vi "Check Action.vi"(6 "HRS Time":dbl, 7 "Values In":dbl[](array[numeric]), 8 "error in (no error)":errorcluster, 11 "Valve in":refnum<class "TimedPWMControl.lvclass">) -> (0 "error out":errorcluster, 1 "Do Action":bool, 2 "Action":T1, 3 "Valve out":refnum<class "TimedPWMControl.lvclass">, 5 "Values":dbl[](array[numeric]))   [LabVIEW 2020, in "VolatusControl.lvlib" / "TimedPWMControl.lvclass"]
uses:
  TimedPWMControl.lvclass
  Valve Action.ctl
  Volatus/MessageQ/MessageQ.lvclass
  TimedPWMControl.lvclass/TimedPWMControl.ctl
  State.ctl
  lv-vecto/Vecto/Channel/Channel.lvclass/Channel.ctl
  lv-vecto/Vecto/Group/Value by Index.vi
  VolatusControl.lvlib
  lv-control/IG PID/PID/PID.lvclass
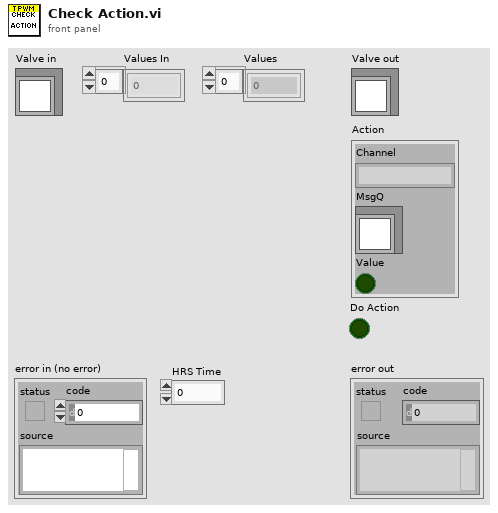
[diagram p1: front panel]
types:
  T1 = typedef "VolatusControl.lvlib/Valve Action.ctl" = cluster{"Channel":string, "MsgQ":refnum<class "MessageQ.lvclass">, "Value":bool}
  T2 = typedef "VolatusControl.lvlib/TimedPWMControl.lvclass/State.ctl" = enum16{"Idle", "Start", "Enabled", "Disable"}
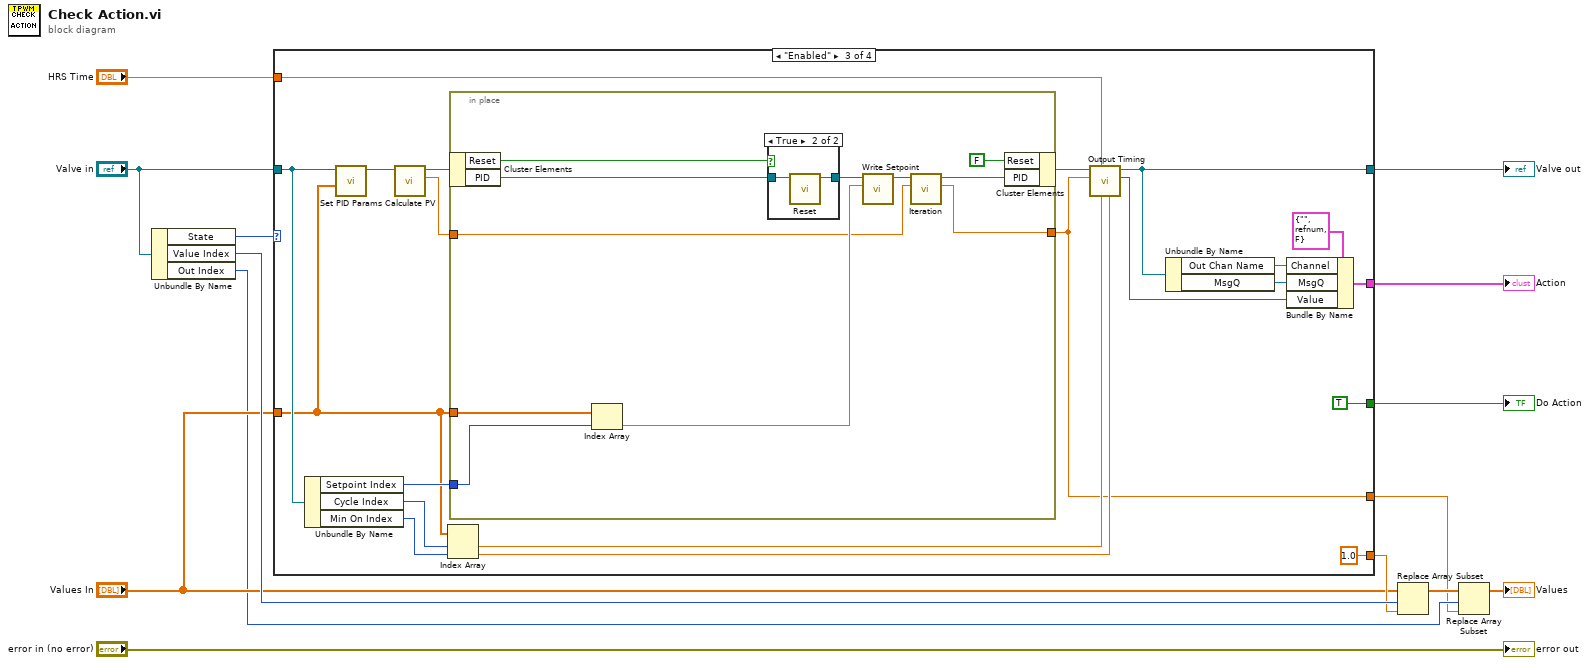
[diagram p0: block diagram]
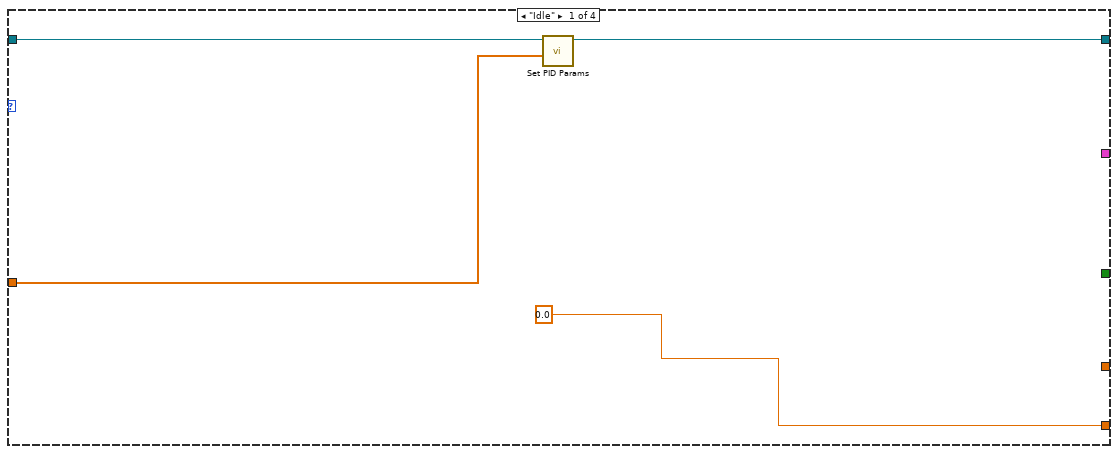
[diagram p2: hidden frame]
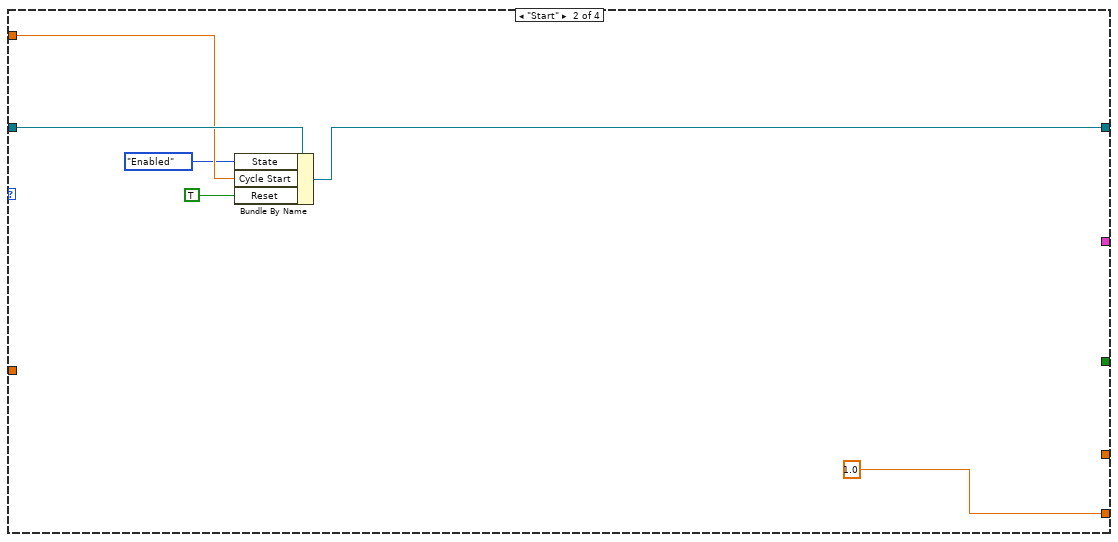
[diagram p3: hidden frame]
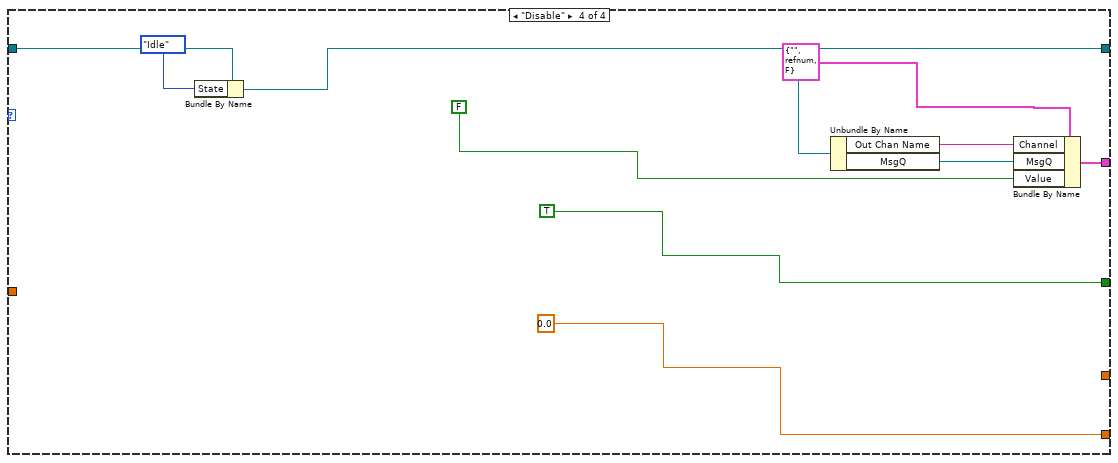
[diagram p5: hidden frame]
diagram:
  n1 = Unbundle By Name("Valve in") -> ("State"=w12:T2, "Value Index"=w13:i32, "Out Index"=w5:i32)
  n2 = case shown="\"Enabled\"" w12 {
    tunnel: [0.0 1.0 1.0 0.0] -> w11
    tunnel: [_ _ TRUE ("Do Action") TRUE ("Do Action")] -> w10
    tunnel: [_ _ w40 w67] -> w9
    tunnel: [w16 w21 w34 w61] -> w8
    tunnel: "Values In" -> [w15 _ w27 _]
    tunnel: [_ _ w31 _] -> w3
    tunnel: "HRS Time" -> [_ w23 w30 _]
    tunnel: "Valve in" -> [w17 w24 w29 w64]
    frame "Idle" {
      n3 = call "Set PID Params.vi"("Values"=w15, "TimedPWMControl in"=w17) -> ("TimedPWMControl out"=w16:refnum<class "TimedPWMControl.lvclass">)  [unwired: 8 in, 1 out]
    }
    frame "Start" {
      n4 = Bundle By Name(cluster=w24, "State"=State."Enabled", "Cycle Start"=w23, "Reset"=TRUE) -> (w21:refnum<class "TimedPWMControl.lvclass">)
    }
    frame "Enabled" {
      n5 = Unbundle By Name(w29) -> ("Setpoint Index"=w41:i32, "Cycle Index"=w39:i32, "Min On Index"=w38:i32)
      n6 = call "Set PID Params.vi"("Values"=w27, "TimedPWMControl in"=w29) -> ("TimedPWMControl out"=w28:refnum<class "TimedPWMControl.lvclass">)  [unwired: 8 in, 1 out]
      n7 = call "Calculate PV.vi"("TimedPWMControl in"=w28) -> ("PV"=w25:dbl, "TimedPWMControl out"=w26:refnum<class "TimedPWMControl.lvclass">)  [unwired: 8 in, 1 out]
      n8 = Index Array(array=w27, index #1=w39, index #2=w38) -> (element #1=w37:dbl, element #2=w36:dbl)
      n9 = in-place {
        in-place-border: w41 -> [w54]
        in-place-border: w27 -> [w55]
        in-place-border: [w51] -> w31
        in-place-border: w25 -> [w46]
        n10 = in-place-cluster #1(w26) -> ("Reset"=w48:bool, "PID"=w47:refnum<class "PID.lvclass">)
        n11 = Index Array(array=w55, index=w54) -> (element=w53:dbl)
        n12 = case shown="True" w48 {
          tunnel: w47 -> [w57 w59]
          tunnel: [w57 w58] -> w49
          frame False {
          }
          frame True {
            n13 = call "Reset.vi"("PID in"=w59) -> ("PID out"=w58:refnum<class "PID.lvclass">)  [unwired: 9 in, 1 out]
          }
        }
        n14 = call "Write Setpoint.vi"("Setpoint"=w53, "PID in"=w49) -> ("PID out"=w56:refnum<class "PID.lvclass">)  [unwired: 8 in, 1 out]
        n15 = call "Iteration.vi"("Process Value"=w46, "PID in"=w56) -> ("Output"=w51:dbl, "PID out"=w52:refnum<class "PID.lvclass">)  [unwired: 6 in, 2 out]
        n16 = in-place-cluster #1("Reset"=FALSE, "PID"=w52) -> (w42:refnum<class "TimedPWMControl.lvclass">)
      }
      n17 = call "Output Timing.vi"("Min On"=w36, "Cycle"=w37, "HRS Time"=w30, "Out 0-1"=w31, "TimedPWMControl in"=w42) -> ("Output"=w35:bool, "TimedPWMControl out"=w34:refnum<class "TimedPWMControl.lvclass">)  [unwired: 4 in, 1 out]
      n18 = Unbundle By Name(w34) -> ("Out Chan Name"=w33:string, "MsgQ"=w32:refnum<class "MessageQ.lvclass">)
      n19 = Bundle By Name(cluster=T1 {"Channel"="", "MsgQ"=refnum, "Value"=FALSE} ("Action"), "Channel"=w33, "MsgQ"=w32, "Value"=w35) -> (w40:T1)
    }
    frame "Disable" {
      n20 = Bundle By Name(cluster=w64, "State"=State."Idle") -> (w61:refnum<class "TimedPWMControl.lvclass">)
      n21 = Unbundle By Name(w61) -> ("Out Chan Name"=w62:string, "MsgQ"=w63:refnum<class "MessageQ.lvclass">)
      n22 = Bundle By Name(cluster=T1 {"Channel"="", "MsgQ"=refnum, "Value"=FALSE} ("Action"), "Channel"=w62, "MsgQ"=w63, "Value"=FALSE) -> (w67:T1)
    }
  }
  "Valve out" <- w8
  "Action" <- w9
  "Do Action" <- w10
  n23 = Replace Array Subset(array="Values In", new element=w11, index=w13) -> (w6:dbl[])
  n24 = Replace Array Subset(array=w6, new element=w3, index=w5) -> (→"Values":dbl[])
  "error out" <- "error in (no error)"
